vi "SubVI_Example_Binning_and_Subsampling.vi"(8 "Error In":errorcluster, 9 "Subsampling Mode":i32, 10 "Binning Mode":i32, 11 ".NET (Reference)":refnum<k24>) -> (0 "Error Out":errorcluster, 1 "Subsampling mode supported":bool, 2 "Binning mode supported":bool)   [LabVIEW 2010]
uses:
  C:/Program Files (x86)/National Instruments/LabVIEW 2016/instr.lib/IDS/ueye.NET/uEyeDotNet.dll
  Program Files (x86)/National Instruments/LabVIEW 2016/instr.lib/IDS/ueye.NET/uEyeDotNet.dll
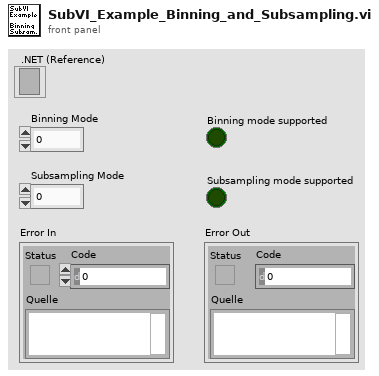
[diagram p1: front panel]
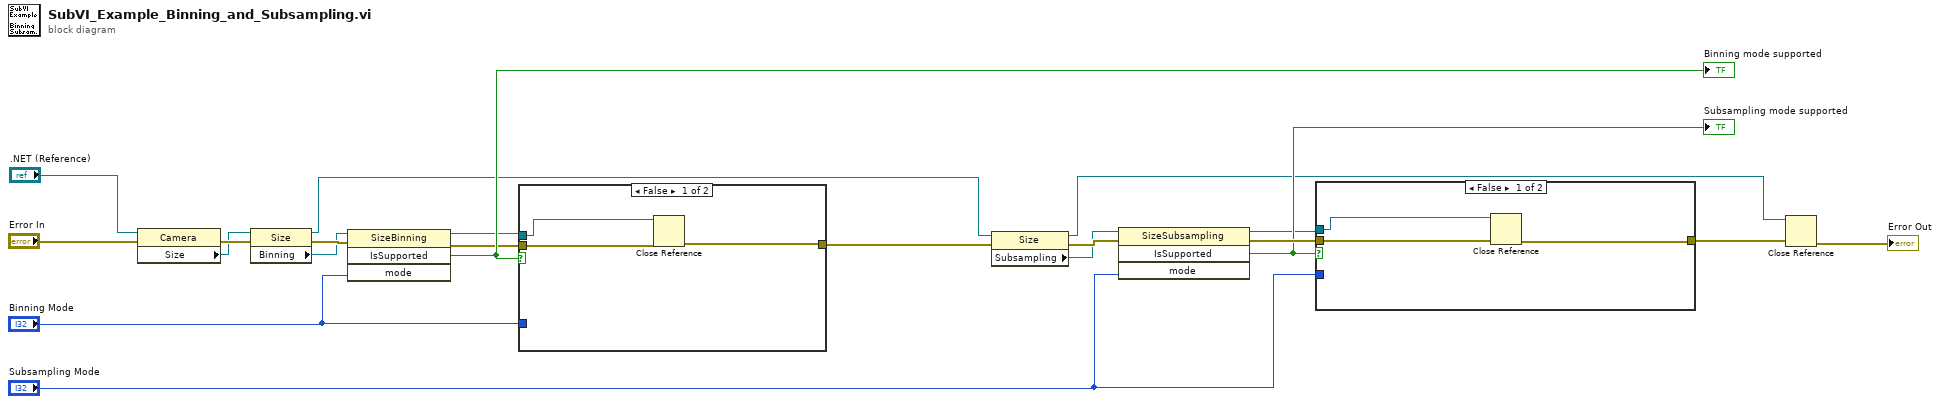
[diagram p0: block diagram]
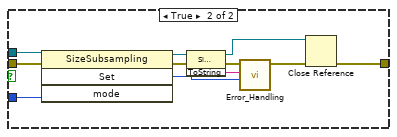
[diagram p2: hidden frame]
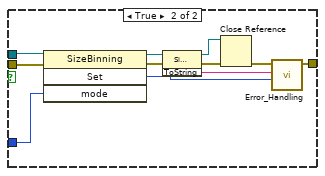
[diagram p3: hidden frame]
diagram:
  n1 = property class="Camera"(reference=".NET (Reference)", error in="Error In") -> (error out=w20:errorcluster, "Size"=w2:refnum<k24>)  [unwired: 1 out]
  n2 = property class="Size"(reference=w2, error in=w20) -> (reference out=w1:refnum<k24>, error out=w18:errorcluster, "Binning"=w9:refnum<k24>)
  n3 = invoke class="SizeBinning" method="IsSupported"(reference=w9, error in=w18, "mode"="Binning Mode") -> (reference out=w8:refnum<k24>, error out=w15:errorcluster, "IsSupported"=w16:bool)  [unwired: 1 in, 1 out]
  "Binning mode supported" <- w16
  n4 = case shown="False" w16 {
    tunnel: [w23 w35] -> w3
    tunnel: "Binning Mode" -> [_ w30]
    tunnel: w15 -> [w24 w29]
    tunnel: w8 -> [w22 w28]
    frame False {
      n5 = Close Reference(reference=w22, error in (no error)=w24) -> (error out=w23:errorcluster)
    }
    frame True {
      n6 = invoke class="SizeBinning" method="Set"(reference=w28, error in=w29, "mode"=w30) -> (reference out=w32:refnum<k24>, error out=w33:errorcluster, "Set"=w34:i32)  [unwired: 1 in, 1 out]
      n7 = invoke class="SizeBinning" method="ToString"(reference=w32, error in=w33) -> (reference out=w25:refnum<k24>, error out=w27:errorcluster, "ToString"=w31:string)  [unwired: 1 in]
      n8 = Close Reference(reference=w25, error in (no error)=w27) -> (error out=w26:errorcluster)
      n9 = call "Error_Handling.vi"("Error Code"=w34, "Error String"=w31, "Error In"=w26) -> ("Error Out"=w35:errorcluster)  [unwired: 8 in]
    }
  }
  n10 = property class="Size"(reference=w1, error in=w3) -> (reference out=w4:refnum<k24>, error out=w14:errorcluster, "Subsampling"=w11:refnum<k24>)
  n11 = invoke class="SizeSubsampling" method="IsSupported"(reference=w11, error in=w14, "mode"="Subsampling Mode") -> (reference out=w5:refnum<k24>, error out=w12:errorcluster, "IsSupported"=w10:bool)  [unwired: 1 in, 1 out]
  "Subsampling mode supported" <- w10
  n12 = case shown="False" w10 {
    tunnel: [w37 w40] -> w7
    tunnel: "Subsampling Mode" -> [_ w44]
    tunnel: w12 -> [w38 w43]
    tunnel: w5 -> [w36 w42]
    frame False {
      n13 = Close Reference(reference=w36, error in (no error)=w38) -> (error out=w37:errorcluster)
    }
    frame True {
      n14 = invoke class="SizeSubsampling" method="Set"(reference=w42, error in=w43, "mode"=w44) -> (reference out=w47:refnum<k24>, error out=w48:errorcluster, "Set"=w49:i32)  [unwired: 1 in, 1 out]
      n15 = invoke class="SizeSubsampling" method="ToString"(reference=w47, error in=w48) -> (reference out=w39:refnum<k24>, error out=w45:errorcluster, "ToString"=w46:string)  [unwired: 1 in]
      n16 = call "Error_Handling.vi"("Error Code"=w49, "Error String"=w46, "Error In"=w45) -> ("Error Out"=w41:errorcluster)  [unwired: 8 in]
      n17 = Close Reference(reference=w39, error in (no error)=w41) -> (error out=w40:errorcluster)
    }
  }
  n18 = Close Reference(reference=w4, error in (no error)=w7) -> (error out=→"Error Out":errorcluster)
